vi "Measure_Synthetic_Jet.vi"(3 "Mode":T1=enum."Run VI", 5 "Traverse line In":T3={"Start X"=0.0, "Start Y"=0.0, "Start Z"=0.0, "End X"=nan, "End Y"=nan, "End Z"=nan, "No. of pts."=5, "Spacing"=enum."Linear", "Filename"=path "C:/EnFlo_Data_Local/2013/Aero_Tunnel/Nick_Martin/Results/01-2013/QA_test_I.xls", "Tunnel Speed"=nan, "Averaging time (min)"=0.08, "Extra Commands"="", "Specific Arguments"="Measure_Synthetic_Jet.vi; 200; 1000; 100", "Emission Rate (l/min)"=nan, "Trace Gas Concentration (%)"=nan, "Density Ratio"="  ---------", "Comments"="", "Row No"=0, "Row Type Selector"=enum."Run VI Named:", "Completion time"="17:12  07-01-2013", "Row Duration (mins)"=4.483248000000001, "No. of Valid pts."=5, "Meas Setup File"="LDA_SJ_A.xls"} {"Row Duration (mins)" format="%#.1f"; "Row No" min=0; "Trace Gas Concentration (%)" min=0.0 format="%#.2f"; "Emission Rate (l/min)" format="%#.2f"; "Tunnel Speed" format="%#.2f"; "Start X" format="%#.2f"; "Start Y" format="%#.2f"; "Start Z" format="%#.2f"; "End X" format="%#.2f"; "End Y" format="%#.2f"; "End Z" format="%#.2f"; "Averaging time (min)" min=0.0 format="%#.2f"}) -> (0 "Error Message":string, 1 "Status":T2, 2 "Traverse line Out":T3={"Start X"=0.0, "Start Y"=0.0, "Start Z"=0.0, "End X"=nan, "End Y"=nan, "End Z"=nan, "No. of pts."=5, "Spacing"=enum."Linear", "Filename"=path "C:/EnFlo_Data_Local/2013/Aero_Tunnel/Nick_Martin/Results/01-2013/QA_test_I.xls", "Tunnel Speed"=nan, "Averaging time (min)"=0.08, "Extra Commands"="", "Specific Arguments"="Measure_Synthetic_Jet.vi; 200; 1000; 100", "Emission Rate (l/min)"=nan, "Trace Gas Concentration (%)"=nan, "Density Ratio"="  ---------", "Comments"="", "Row No"=0, "Row Type Selector"=enum."Run VI Named:", "Completion time"="17:12  07-01-2013", "Row Duration (mins)"=4.483248000000001, "No. of Valid pts."=5, "Meas Setup File"="LDA_SJ_A.xls"} {"Row Duration (mins)" format="%#.1f"; "Row No" min=0; "Trace Gas Concentration (%)" min=0.0 format="%#.2f"; "Emission Rate (l/min)" format="%#.2f"; "Tunnel Speed" format="%#.2f"; "Start X" format="%#.2f"; "Start Y" format="%#.2f"; "Start Z" format="%#.2f"; "End X" format="%#.2f"; "End Y" format="%#.2f"; "End Z" format="%#.2f"; "Averaging time (min)" min=0.0 format="%#.2f"})   [LabVIEW 2011]
uses:
  Gen Trav/Traverse_cluster.ctl
  Gen Trav/Spacing.ctl
  Controls/Multi_run_mode.ctl
  Gen Trav/Multi_Run_Status.ctl
  Controls/User_Specific_mode.ctl
  Controls/Save_Data.ctl
  Controls/Setup.ctl
  ADAM Client/Sub VIs/ADAM Controls/Update_scan_value.ctl
  Globals/Synthetic_jet_global.vi
  <vilib>/Analysis/1siggen.llb/Ramp Pattern by Samples.vi
  Globals/Extra_Commands_Global.vi
  Globals/Meas_global.vi
  <vilib>/Analysis/NI_AALBase.lvlib
panel:
  in  "Stop Button":bool
  out "Last Meas Point":bool=TRUE
  out "Data":cluster{"Ramp Pattern":dbl[], dbl[]}[](graph)
  in  "Channels to Analyse":i32[](listbox)=[0]
  in  "VISA resource name":refnum<visa-resource-name>="USB0::0x0699::0x0347::C036837::INSTR"
  out "First Meas Point":bool=TRUE
  # "Check the Multirun in order to populate these Channels!"
  # "X           Y            Z"
  # "Start"
  # "End"
  # "X           Y            Z"
  # "Start"
  # "End"
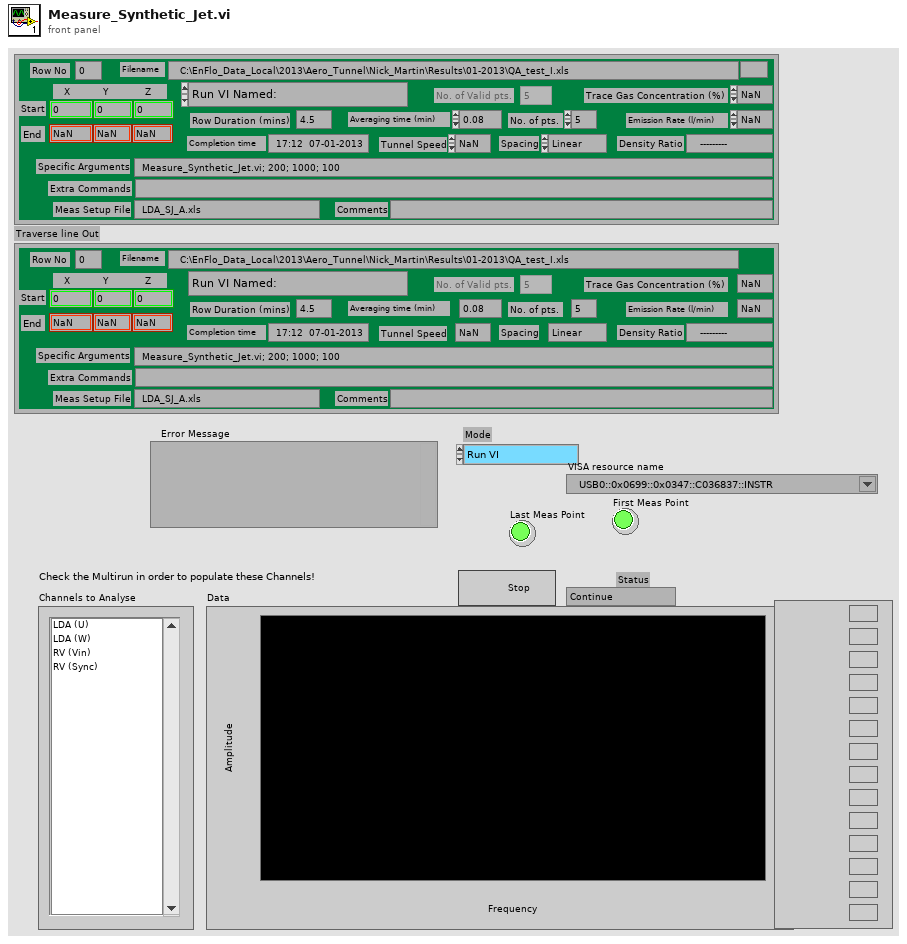
[diagram p1: front panel]
types:
  T1 = typedef "User_Specific_mode.ctl" = enum16{"Check VI only", "Run VI"}
  T2 = typedef "Multi_Run_Status.ctl" = enum16{"Continue", "Jump to Next Point", "Jump to Next Row", "Jump To Fall Back", "Terminate Run"}
  T3 = typedef "Traverse_cluster.ctl" = cluster{"Start X":dbl, "Start Y":dbl, "Start Z":dbl, "End X":dbl, "End Y":dbl, "End Z":dbl, "No. of pts.":i32, "Spacing":T4, "Filename":path, "Tunnel Speed":dbl, "Averaging time (min)":dbl, "Extra Commands":string, "Specific Arguments":string, "Emission Rate (l/min)":dbl, "Trace Gas Concentration (%)":dbl, "Density Ratio":string, "Comments":string, "Row No":i32, "Row Type Selector":T5, "Completion time":string, "Row Duration (mins)":dbl, "No. of Valid pts.":i32, "Meas Setup File":string}
  T4 = typedef "Spacing.ctl" = enum16{"Linear", "Log", "Gauss", "Specified", "N/A"}
  T5 = typedef "Multi_run_mode.ctl" = enum16{"Move Traverse Only", "Set Tunnel Speed Only", "Set Source Only", "Set Measurement Conditions", "Single Measurement", "Vertical Profile", "Lateral Profile", "Longitudinal Profile", "Explore Volume", "Multi-Axis Profile", "Auto Calibrate", "Meas Fast FID Bkgnd", "Check Beam Power", "Scanning Valve Measurement", "Run VI Named:", "Set ADAM Ch", "Wait (minutes)", "Send Message", "Synchronize With:", "Fall Back to this Row", "Turn Off Row Repeating", "Blank Row", "Traverse 3D Volume"}
  T6 = typedef "Save_Data.ctl" = enum16{"Save No Data", "Save Data"}
  T7 = typedef "Setup.ctl" = enum16{"Run Program", "Show Setup", "Save Current Setup", "Setup Front Panel"}
  T8 = typedef "SJ_Data_Cluster.ctl" = cluster{"Do (mm)":dbl, "Dc (mm)":dbl, "Ho (mm)":dbl, "Hc (mm)":dbl, "K":dbl, "beta":dbl, "Vc (m^3)":dbl, "Vo (m^3)":dbl}
  T9 = typedef "Update_scan_value.ctl" = cluster{"Channel Name":string, "New Value":dbl}
  T10 = typedef "Analysis_info_cluster.ctl" = cluster{"Colour":u32, "Inst type":T11, "Inst name":string, "Symbol":string, "Code name":string, "Extra Info":string, "Inst Array":T12, "Extra Titles":string[], "Extra Values":string[], "U":dbl, "u^2":dbl, "u^3":dbl, "u^4":dbl, "Skew_u":dbl, "Kurt_u":dbl, "Sd Error in Mean":dbl, "% u'/U":dbl, "X":dbl, "Y":dbl, "Z":dbl, "Timescale integral to 25%":dbl, "Sd Error in Variance":dbl, "Calib File":path, "Calib Constants":dbl[], "Output Position":bool, "Full Stats":bool, "Av Sampling Rate":dbl, "Av No of Samples":dbl, "Total Meas Time (s)":dbl, "ADAM Ch Name":string}
  T11 = typedef "Inst_type.ctl" = enum16{"Propeller anemometer", "Raw voltage", "Pressure Transducer", "Pitot-static tube", "Preston tube", "Hot wire", "Cross wire 1", "Cross wire 2", "Generic Linear", "Generic Polynomial", "Generic BackPoly", "Fast FID", "Thermocouple", "Cold wire", "Pulsed Wire", "LDA Vel", "LDA Tran time", "LDA Arr time"}
  T12 = typedef "Instrument_Array.ctl" = enum16{"PWA", "LDA", "Analogue"}
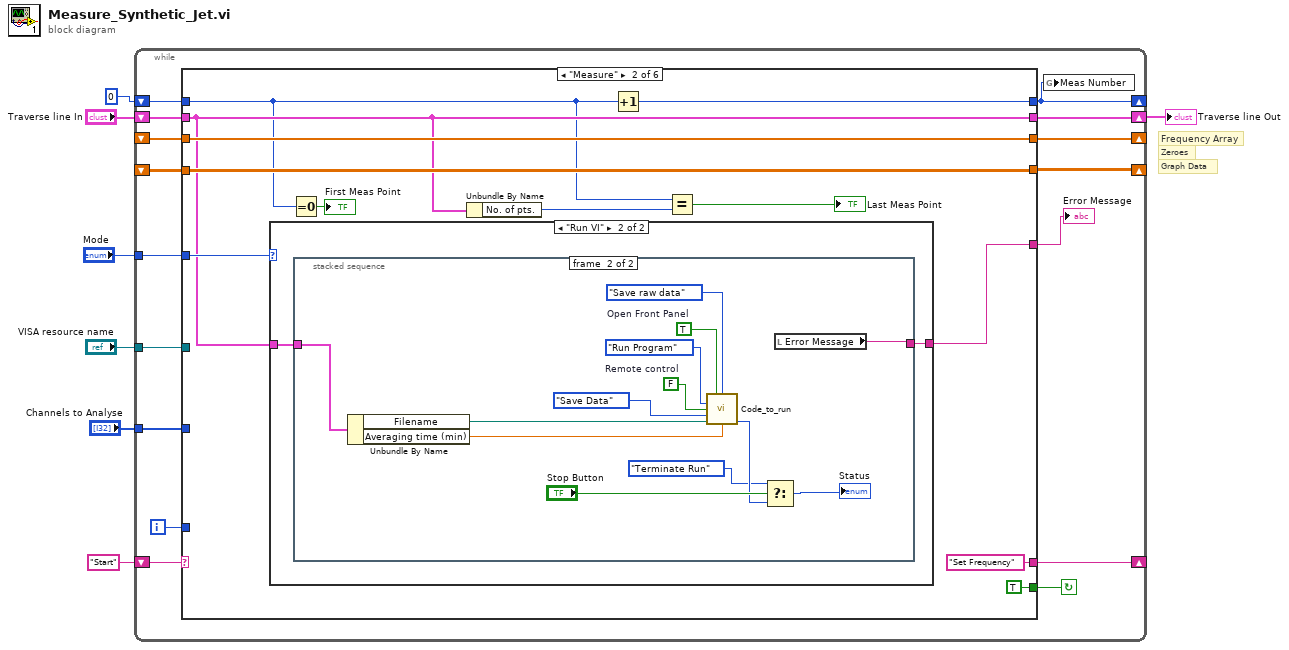
[diagram p0: block diagram]
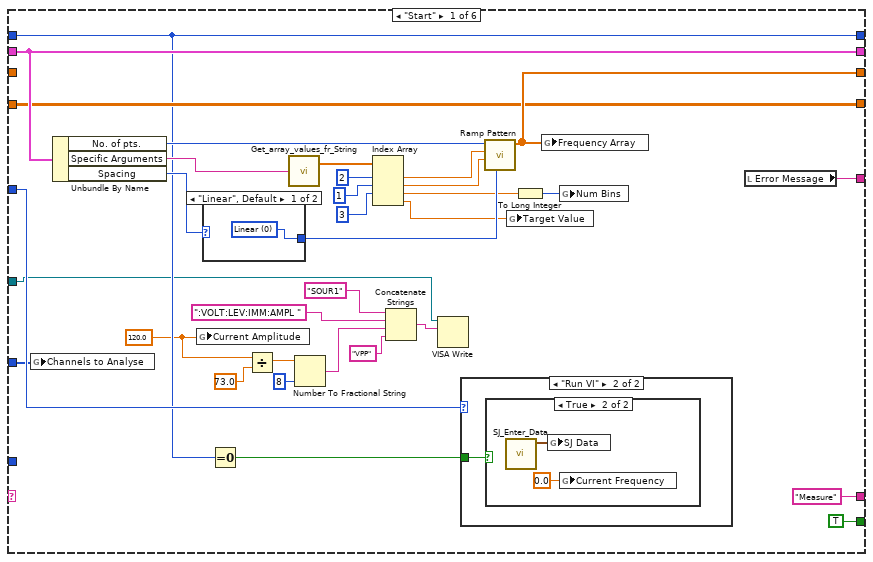
[diagram p2: hidden frame]
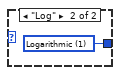
[diagram p5: hidden frame]
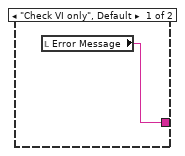
[diagram p6: hidden frame]
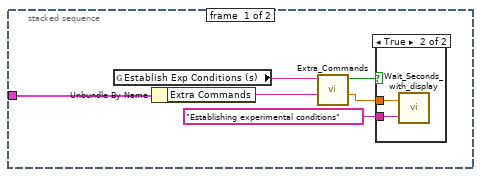
[diagram p7: hidden frame]
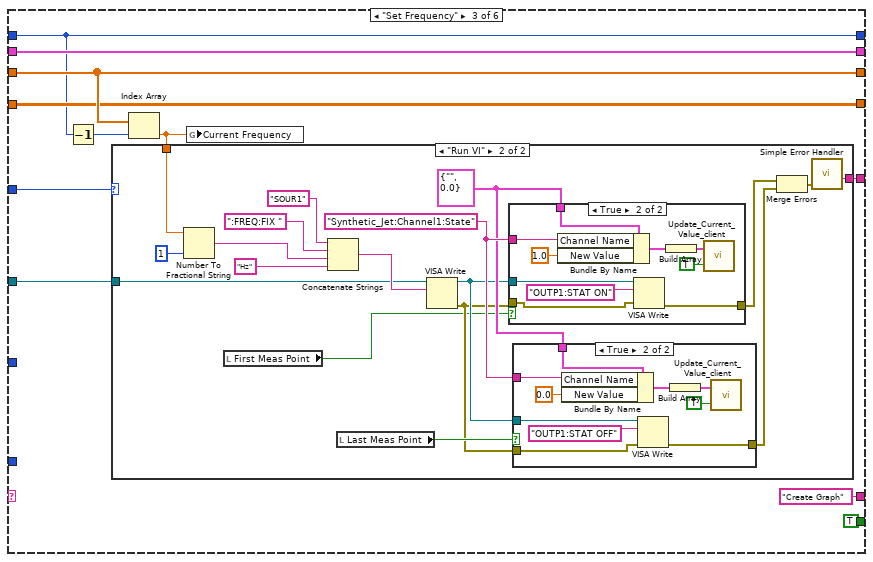
[diagram p9: hidden frame]
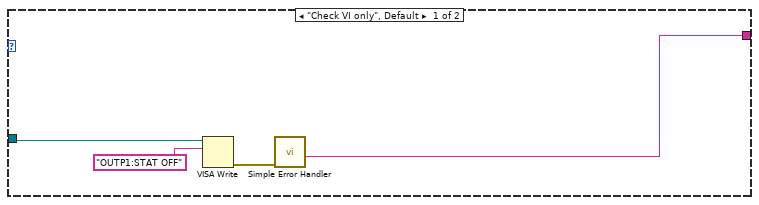
[diagram p10: hidden frame]
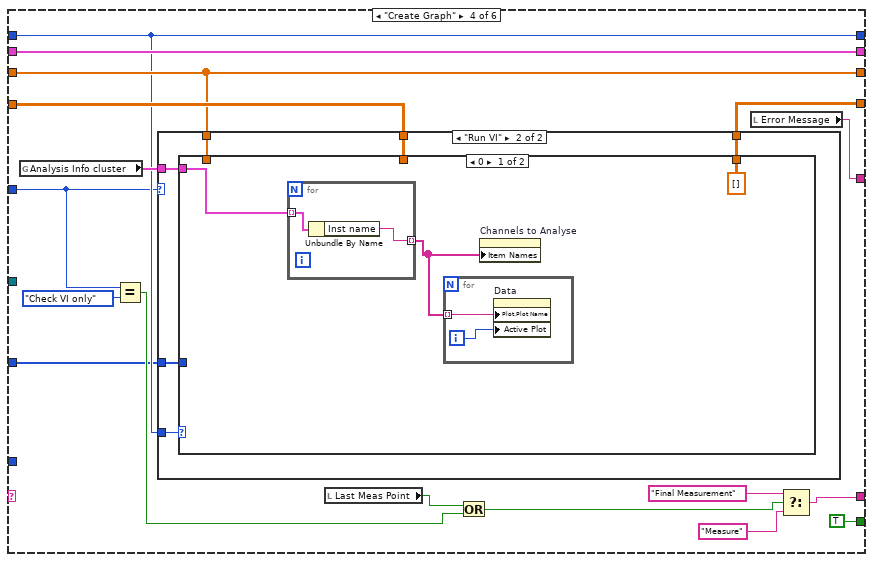
[diagram p13: hidden frame]
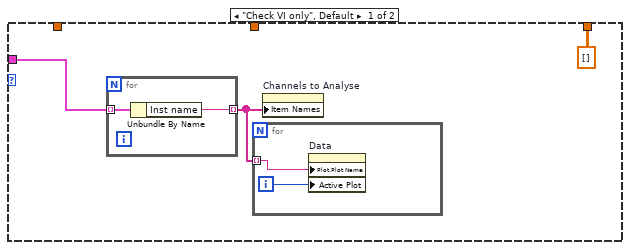
[diagram p14: hidden frame]
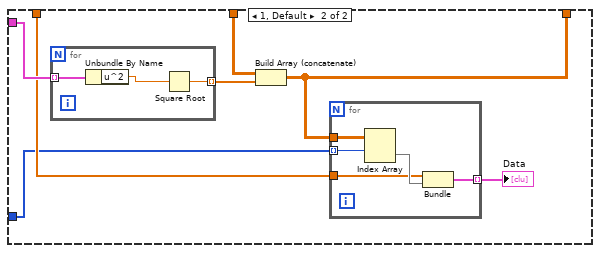
[diagram p15: hidden frame]
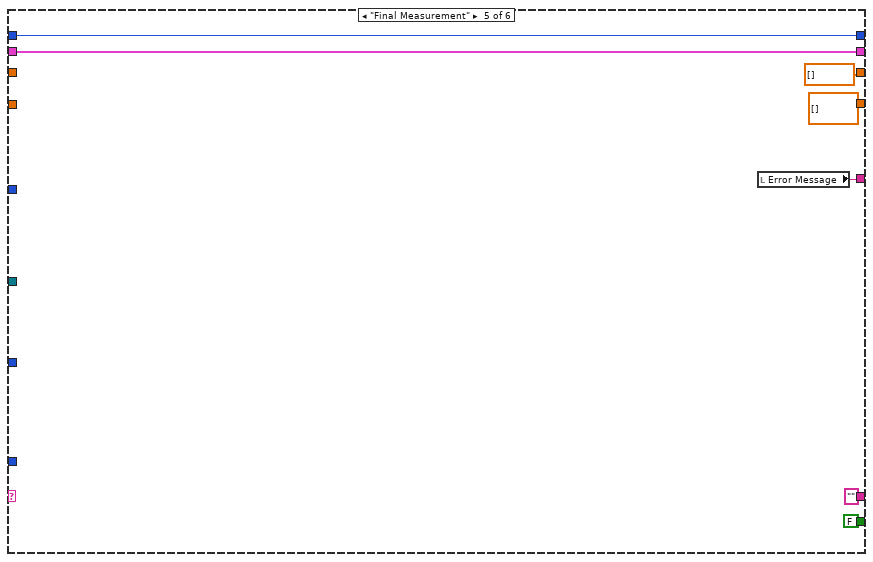
[diagram p16: hidden frame]
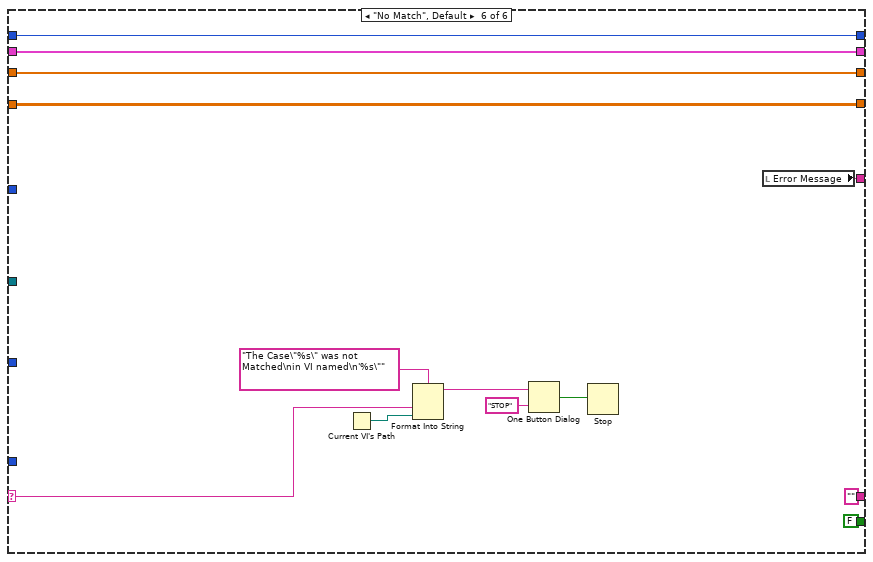
[diagram p17: hidden frame]
diagram:
  # "Graph Data"
  # "Zeroes"
  # "Frequency Array"
  n1 = while {
    shift-right: [w21] -> _
    shift-left: "Start" -> [w20]
    shift-right: [w19] -> w5
    shift-left: "Traverse line In" -> [w23]
    shift-right: [w18] -> _
    shift-left: _ -> [w17]
    tunnel: "Mode" -> [w16]
    tunnel: "VISA resource name" -> [w14]
    shift-right: [w13] -> _
    shift-left: _ -> [w12]
    shift-right: [w9] -> _
    shift-left: 0 -> [w10]
    tunnel: "Channels to Analyse" -> [w8]
    i -> [w15]
    stop <- w22 continue-if-true
    n2 = case shown="\"Measure\"" w20 {
      selector: w20 -> [_ _ _ _ _ w216]
      tunnel: w23 -> [w54 w66 w106 w169 w209 w224]
      tunnel: [TRUE TRUE TRUE TRUE ("Last Meas Point") FALSE ("Last Meas Point") FALSE] -> w22
      tunnel: ["Measure" "Set Frequency" "Create Graph" w162 "" ""] -> w21
      tunnel: [w54 w66 w106 w169 w209 w224] -> w19
      tunnel: [w42 w71 w105 w165 dbl[] [] ("Ramp Pattern") w215] -> w18
      tunnel: w17 -> [_ w71 w105 w165 _ w215]
      tunnel: w16 -> [w43 w70 w101 w158 _ _]
      tunnel: w15 -> [_ _ _ _ _ _]
      tunnel: w14 -> [w27 _ w102 _ _ _]
      tunnel: [w41 w69 w100 w167 dbl[][] [] w214] -> w13
      tunnel: w12 -> [w41 w69 w100 w166 _ w214]
      tunnel: [w40 w68 w99 w164 w208 w213] -> w11
      tunnel: [w36 w64 w98 w159 w205 w212] -> w9
      tunnel: w10 -> [w36 w62 w98 w159 w205 w212]
      tunnel: w8 -> [w35 _ _ w153 _ _]
      frame "Start" {
        w24 = 120.0 ("number")
        n3 = global write "Synthetic_jet_global.vi" "Channels to Analyse"(w35) -> ()
        n4 = Unbundle By Name(w54) -> ("No. of pts."=w53:i32, "Specific Arguments"=w50:string, "Spacing"=w52:T4)
        n5 = global write "Synthetic_jet_global.vi" "Current Amplitude"(w24) -> ()
        n6 = case shown="\"Linear\", Default" w52 {
          tunnel: [w60 w61] -> w51
          frame "Linear", Default {
            w60 = u16 0 items=["Linear", "Logarithmic"] ("type")
          }
          frame "Log" {
            w61 = u16 1 items=["Linear", "Logarithmic"] ("type")
          }
        }
        n7 = Equal To 0?(x=w36) -> (x = 0?=w44:bool)
        n8 = Divide(x=w24, y=73.0) -> (x/y=w26:dbl)
        n9 = call "Get_array_values_fr_String.vi"("String Value"=w50) -> ("Numeric Array"=w49:dbl[])  [unwired: 1 out]
        n10 = Number To Fractional String(number=w26, precision (6)=i16 8) -> (F-format string=w29:string)  [unwired: 2 in]
        n11 = Index Array(array=w49, index #1=2 ("index"), index #2=1 ("index"), index #3=3 ("index")) -> (element #1=w46:dbl, element #2=w45:dbl, element #3=w38:dbl, element #4=w34:dbl)  [unwired: 1 in]
        n12 = Concatenate Strings("SOUR1" ("string"), ":VOLT:LEV:IMM:AMPL " ("string"), w29, "VPP" ("string")) -> (w30:string)
        n13 = VISA Write(VISA resource name=w27, write buffer=w30) -> ()  [unwired: 1 in, 3 out]
        n14 = case shown="\"Run VI\"" w43 {
          tunnel: w44 -> [_ w57]
          frame "Check VI only", Default {
          }
          frame "Run VI" {
            n15 = case shown="True" w57 {
              frame False {
              }
              frame True {
                n16 = call "SJ_Enter_Data.vi"() -> ("SJ Data"=w59:T8)  [unwired: 11 in]
                n17 = global write "Synthetic_jet_global.vi" "SJ Data"(w59) -> ()
                n18 = global write "Synthetic_jet_global.vi" "Current Frequency"(0.0 ("Current Frequency")) -> ()
              }
            }
          }
        }
        n19 = call-poly <vilib>:"Ramp Pattern.vi"("type"=w51, "start"=w45, "end"=w46, "samples"=w53) -> ("Ramp Pattern"=w42:dbl[])  [unwired: 6 in, 1 out]
        n20 = global write "Synthetic_jet_global.vi" "Target Value"(w34) -> ()
        n21 = To Long Integer(number=w38) -> (32bit integer=w37:i32)
        n22 = global write "Synthetic_jet_global.vi" "Frequency Array"(w42) -> ()
        n23 = global write "Synthetic_jet_global.vi" "Num Bins"(w37) -> ()
        n24 = local read "Error Message"() -> (w40:string)
      }
      frame "Measure" {
        n25 = case shown="\"Run VI\"" w70 {
          tunnel: w66 -> [_ w76]
          tunnel: [w74 w75] -> w68
          frame "Check VI only", Default {
            n26 = local read "Error Message"() -> (w74:string)
          }
          frame "Run VI" {
            n27 = stacked-sequence {
              tunnel: w76 -> [w77 w93]
              tunnel: [_ w90] -> w75
              frame #0 {
                n28 = global read "Extra_Commands_Global.vi" "Establish Exp Conditions (s)"() -> (w80:string)
                n29 = Unbundle By Name(w77) -> ("Extra Commands"=w78:string)
                n30 = call "Extra_Commands.vi"("String to Search"=w78, "Command"=w80) -> ("Numeric Value"=w79:dbl, "Command Found"=w81:bool)  [unwired: 2 in, 2 out]
                n31 = case shown="True" w81 {
                  tunnel: w79 -> [_ w84]
                  tunnel: "Establishing experimental conditions" ("Message") -> [_ w83]
                  frame False {
                  }
                  frame True {
                    n32 = call "Wait_Seconds_with_display.vi"("Message"=w83, "Seconds to wait"=w84) -> ()  [unwired: 1 in, 1 out]
                  }
                }
              }
              frame #1 {
                w95 = TRUE  # Open Front Panel
                w94 = FALSE  # Remote control
                n33 = Unbundle By Name(w93) -> ("Filename"=w92:path, "Averaging time (min)"=w89:dbl)
                n34 = call "Code_to_run.vi"("Open Front Panel"=w95, "Raw data option"=enum16{"Save raw data", "Raw data not saved"}."Save raw data", "setup"=Setup."Run Program", "Remote control"=w94, "File"=Save_Data."Save Data", "Results Filename"=w92, "Averaging time (min)"=w89) -> ("Status"=w87:T2)  [unwired: 4 in, 4 out]
                n35 = Select(t=Multi_Run_Status."Terminate Run", s="Stop Button", f=w87) -> (s? t:f=→"Status":T2)
                n36 = local read "Error Message"() -> (w90:string)
              }
            }
          }
        }
        n37 = Equal To 0?(x=w62) -> (x = 0?=→"First Meas Point":bool)
        n38 = Unbundle By Name(w66) -> ("No. of pts."=w65:i32)
        n39 = Increment(x=w62) -> (x+1=w64:i32)
        n40 = Equal?(x=w62, y=w65) -> (x = y?=→"Last Meas Point":bool)
      }
      frame "Set Frequency" {
        n41 = Decrement(x=w98) -> (x-1=w104:i32)
        n42 = Index Array(array=w105, index=w104) -> (element=w103:dbl)
        n43 = case shown="\"Run VI\"" w101 {
          tunnel: w103 -> [_ w122]
          tunnel: w102 -> [w111 w121]
          tunnel: [w109 w118] -> w99
          frame "Check VI only", Default {
            n44 = VISA Write(VISA resource name=w111, write buffer="OUTP1:STAT OFF") -> (error out=w110:errorcluster)  [unwired: 1 in, 2 out]
            n45 = call <vilib>:"Simple Error Handler.vi"("error in (no error)"=w110) -> ("source out"=w109:string)  [unwired: 4 in, 4 out]
          }
          frame "Run VI" {
            w123 = T9 {"Channel Name"="", "New Value"=0.0} ("Update Scan Value Cluster")
            w124 = "Synthetic_Jet:Channel1:State" ("write buffer")
            n46 = Number To Fractional String(number=w122, precision (6)=i16 1) -> (F-format string=w128:string)  [unwired: 2 in]
            n47 = local read "First Meas Point"() -> (w113:bool)
            n48 = Concatenate Strings("SOUR1", ":FREQ:FIX " ("string"), w128, "Hz" ("string")) -> (w130:string)
            n49 = local read "Last Meas Point"() -> (w120:bool)
            n50 = VISA Write(VISA resource name=w121, write buffer=w130) -> (VISA resource name out=w119:refnum<visa-resource-name>, error out=w114:errorcluster)  [unwired: 1 in, 1 out]
            n51 = case shown="True" w113 {
              tunnel: w124 -> [_ w147]
              tunnel: w123 -> [_ w146]
              tunnel: w119 -> [_ w145]
              tunnel: [w142 w144] -> w115
              tunnel: w114 -> [w142 w143]
              frame False {
              }
              frame True {
                n52 = Bundle By Name(cluster=w146, "Channel Name"=w147, "New Value"=1.0) -> (w150:T9)
                n53 = VISA Write(VISA resource name=w145, write buffer="OUTP1:STAT ON", error in (no error)=w143) -> (error out=w144:errorcluster)  [unwired: 2 out]
                n54 = Build Array(w150) -> (w149:T9[])
                n55 = call "Update_Current_Value_client.vi"("Don't Bother with check?"=TRUE, "Update array in"=w149) -> ()
              }
            }
            n56 = case shown="True" w120 {
              tunnel: w124 -> [_ w136]
              tunnel: w123 -> [_ w135]
              tunnel: w119 -> [_ w134]
              tunnel: [w131 w133] -> w116
              tunnel: w114 -> [w131 w132]
              frame False {
              }
              frame True {
                n57 = Bundle By Name(cluster=w135, "Channel Name"=w136, "New Value"=0.0) -> (w139:T9)
                n58 = VISA Write(VISA resource name=w134, write buffer="OUTP1:STAT OFF", error in (no error)=w132) -> (error out=w133:errorcluster)  [unwired: 2 out]
                n59 = Build Array(w139) -> (w138:T9[])
                n60 = call "Update_Current_Value_client.vi"("Don't Bother with check?"=TRUE, "Update array in"=w138) -> ()
              }
            }
            n61 = Merge Errors(w115, w116) -> (w117:errorcluster)
            n62 = call <vilib>:"Simple Error Handler.vi"("error in (no error)"=w117) -> ("source out"=w118:string)  [unwired: 4 in, 4 out]
          }
        }
        n63 = global write "Synthetic_jet_global.vi" "Current Frequency"(w103) -> ()
      }
      frame "Create Graph" {
        n64 = global read "Meas_global.vi" "Analysis Info cluster"() -> (w168:T10[])
        n65 = Equal?(x=w158, y=User_Specific_mode."Check VI only") -> (x = y?=w155:bool)
        n66 = case shown="\"Run VI\"" w158 {
          tunnel: w168 -> [w172 w182]
          tunnel: w159 -> [_ w181]
          tunnel: [dbl[][] [] w180] -> w167
          tunnel: w166 -> [_ w179]
          tunnel: w165 -> [_ w178]
          tunnel: w153 -> [_ w177]
          frame "Check VI only", Default {
            n67 = for {
              tunnel: w172 -> [w176] mode=indexing
              tunnel: [w175] -> w170 mode=indexing
              n68 = Unbundle By Name(w176) -> ("Inst name"=w175:string)
            }
            n69 = for {
              tunnel: w170 -> [w174] mode=indexing
              i -> [w173]
              n70 = property on="Data" class="XYGraph (strict)"("Plot.Plot Name"=w174, "Active Plot"=w173) -> ()  [unwired: 2 in, 2 out]
            }
            n71 = property on="Channels to Analyse" class="LstBox (strict)"("Item Names"=w170) -> ()  [unwired: 2 in, 2 out]
          }
          frame "Run VI" {
            n72 = case shown="0" w181 {
              tunnel: w182 -> [w185 w196]
              tunnel: [dbl[][] [] w193] -> w180
              tunnel: w179 -> [_ w194]
              tunnel: w178 -> [_ w192]
              tunnel: w177 -> [_ w190]
              frame 0 {
                n73 = for {
                  tunnel: w185 -> [w189] mode=indexing
                  tunnel: [w188] -> w183 mode=indexing
                  n74 = Unbundle By Name(w189) -> ("Inst name"=w188:string)
                }
                n75 = for {
                  tunnel: w183 -> [w187] mode=indexing
                  i -> [w186]
                  n76 = property on="Data" class="XYGraph (strict)"("Plot.Plot Name"=w187, "Active Plot"=w186) -> ()  [unwired: 2 in, 2 out]
                }
                n77 = property on="Channels to Analyse" class="LstBox (strict)"("Item Names"=w183) -> ()  [unwired: 2 in, 2 out]
              }
              frame 1, Default {
                n78 = for {
                  tunnel: w196 -> [w204] mode=indexing
                  tunnel: [w202] -> w195 mode=indexing
                  n79 = Unbundle By Name(w204) -> ("u^2"=w203:dbl)
                  n80 = Square Root(x=w203) -> (sqrt(x)=w202:dbl)
                }
                n81 = Build Array (concatenate)(w194, w195) -> (w193:dbl[][])
                n82 = for {
                  tunnel: w193 -> [w201]
                  tunnel: w190 -> [w200] mode=indexing
                  tunnel: w192 -> [w198]
                  tunnel: [w197] -> w191 mode=indexing
                  n83 = Index Array(array=w201, index (row)=w200) -> (element=w199:dbl[])  [unwired: 1 in]
                  n84 = Bundle("Ramp Pattern"=w198, w199) -> (w197:cluster{"Ramp Pattern":dbl[], dbl[]})  [unwired: 1 in]
                }
                "Data" <- w191
              }
            }
          }
        }
        n85 = local read "Last Meas Point"() -> (w156:bool)
        n86 = Or(x=w156, y=w155) -> (x .or. y?=w154:bool)
        n87 = local read "Error Message"() -> (w164:string)
        n88 = Select(t="Final Measurement", s=w154, f="Measure") -> (s? t:f=w162:string)
      }
      frame "Final Measurement" {
        n89 = local read "Error Message"() -> (w208:string)
      }
      frame "No Match", Default {
        n90 = Current VI's Path() -> (path=w221:path)
        n91 = Format Into String(format string="The Case\"%s\" was not Matched\nin VI named\n'%s\"" ("Format String"), w216, w221) -> (resulting string=w218:string)  [unwired: 2 in, 1 out]
        n92 = One Button Dialog(message=w218, button name ("OK")="STOP") -> (true=w220:bool)
        n93 = Stop(stop? (T)=w220) -> ()
        n94 = local read "Error Message"() -> (w213:string)
      }
    }
    "Error Message" <- w11
    n95 = global write "Synthetic_jet_global.vi" "Meas Number"(w9) -> ()
  }
  "Traverse line Out" <- w5
